vi "WRP Get Element Voltage.vi"(8 "error in (no error)":errorcluster, 11 "elementName":string) -> (0 "error out":errorcluster, 2 "function return":i32, 3 "voltage":dbl)   [LabVIEW 2018, in "SesWrapper.lvlib"]
doc: "int STDCALL WRP_GetElementVoltage(const String elementName, double *voltage);"
uses:
  SesWrapper.lvlib
  build/Debug/SESWrapper.dll
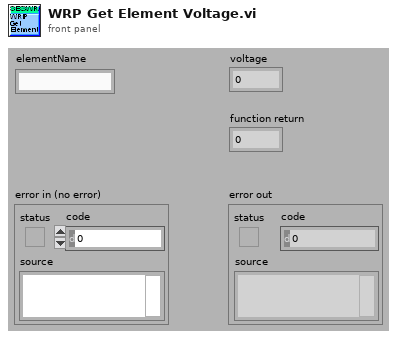
[diagram p1: front panel]
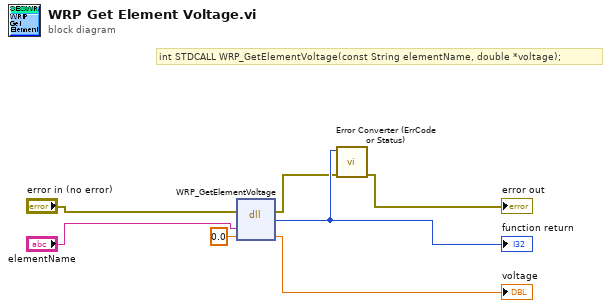
[diagram p0: block diagram]
diagram:
  # "int STDCALL WRP_GetElementVoltage(const String elementName, double *voltage);"
  n1 = dll-call lib="C:/Development/svn/seswrapper-lib/build/Debug/SESWrapper.*" fn="WRP_GetElementVoltage"(error in="error in (no error)", "elementName"="elementName", "voltage"=0.0) -> (error out=w2:errorcluster, w7:i32, "voltage"=→"voltage":dbl)  [unwired: 3 in, 1 out]
  "function return" <- w7
  n2 = call "Error Converter (ErrCode or Status).vi"("error in (no error)"=w2, "error code"=w7) -> ("error out"=→"error out":errorcluster)  [unwired: 9 in]
